vi "Configure Display Bar Graph.vi"(8 "error in (no error)":errorcluster, 9 "graph mode":u16(ring) items=["off", "full scale", "full scale, high level", "full scale, setpoint", "decade", "decade, high level", "decade setpoint", "f(t), 0.2 s/pixel", "f(t), 1 s/pixel", "f(t), 6 s/pixel", "f(t), 1 min./pixel"], 10 "channel":u16(ring) items=["channel 1", "channel 2", "channel 3"], 11 "VGC in":refnum<class "PL Inficon VGC.lvclass">) -> (0 "error out":errorcluster, 1 "graph mode":u16(ring) items=["off", "full scale", "full scale, high level", "full scale, setpoint", "decade", "decade, high level", "decade setpoint", "f(t), 0.2 s/pixel", "f(t), 1 s/pixel", "f(t), 6 s/pixel", "f(t), 1 min./pixel"], 2 "channel":u16(ring) items=["channel 1", "channel 2", "channel 3"], 3 "VGC out":refnum<class "PL Inficon VGC.lvclass">)   [LabVIEW 2015, in "PL Inficon VGC.lvclass"]
doc: "Configures display bar graph."
uses:
  PL Inficon VGC.lvclass
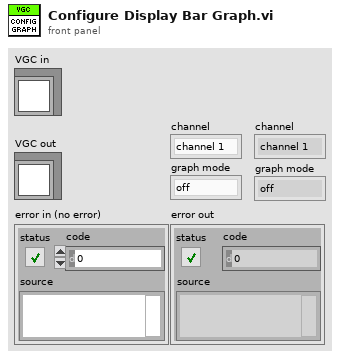
[diagram p1: front panel]
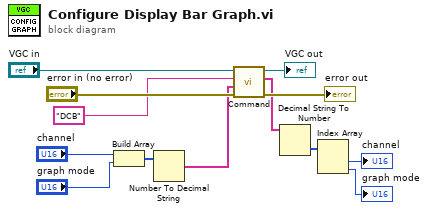
[diagram p0: block diagram]
diagram:
  n1 = Build Array("channel", "graph mode") -> (w7:u16[])
  n2 = Number To Decimal String(number=w7) -> (decimal integer string=w2:string[])  [unwired: 1 in]
  n3 = call "Command.vi"("error in (no error)"="error in (no error)", "parameters"=w2, "command"="DCB" ("format string"), "VGC in"="VGC in") -> ("error out"=→"error out":errorcluster, "response data"=w5:string[], "VGC out"=→"VGC out":refnum<class "PL Inficon VGC.lvclass">)  [unwired: 5 in]
  n4 = Decimal String To Number(string=w5) -> (number=w8:i32[])  [unwired: 2 in, 1 out]
  n5 = Index Array(array=w8) -> (element #1=→"channel":i32, element #2=→"graph mode":i32)  [unwired: 2 in]
